vi "String - String to Bytes (Swapped).vi"(11 "String":string) -> (3 "Sting Out":string)   [LabVIEW 2013]
panel:
  out "unsigned byte array":u8[](array[numeric])
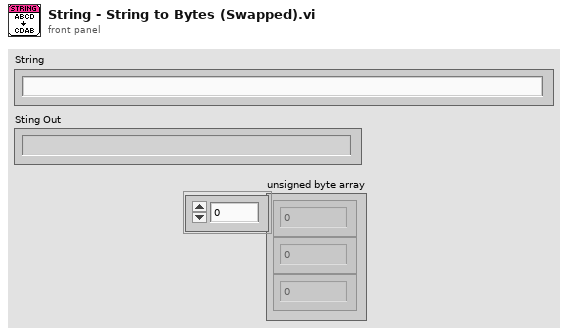
[diagram p1: front panel]
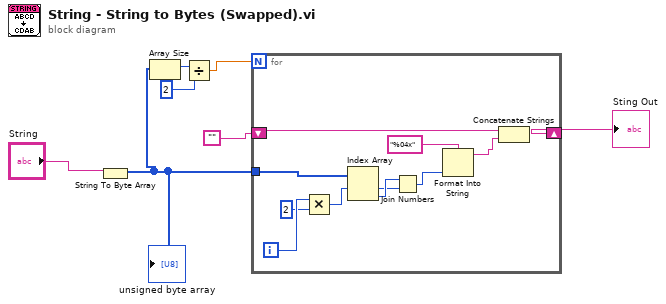
[diagram p0: block diagram]
diagram:
  n1 = String To Byte Array(string="String") -> (unsigned byte array=w4:u8[])
  "unsigned byte array" <- w4
  n2 = Array Size(array=w4) -> (size(s)=w5:i32)
  n3 = Divide(x=w5, y=2) -> (x/y=w2:dbl)
  n4 = for {
    N: w2 -> [_]
    tunnel: w4 -> [w14]
    shift-right: [w17] -> w6
    shift-left: "" -> [w16]
    i -> [w10]
    n5 = Multiply(x=w10, y=2) -> (x*y=w8:i32)
    n6 = Index Array(array=w14, index #1=w8) -> (element #1=w12:u8, element #2=w13:u8)  [unwired: 1 in]
    n7 = Join Numbers(hi=w13, lo=w12) -> ((hi.lo)=w11:u16)
    n8 = Format Into String(format string="%04x", w11) -> (resulting string=w18:string)  [unwired: 2 in, 1 out]
    n9 = Concatenate Strings(w16, w18) -> (w17:string)
  }
  "Sting Out" <- w6
